vi "ADIS16470 Status.vi"(8 "error in (no error)":errorcluster, 11 "ADIS16470DevRef":T1) -> (0 "error out":errorcluster, 2 "ADIS16470 Status":T6, 3 "ADIS16470DevRef":T1)   [LabVIEW 2018]
uses:
  Typedef/ADIS16470 Status.ctl
  Typedef/ADIS16470 Device Reference.ctl
  Typedef/ADIS16470 Hardware Configuration.ctl
  <vilib>/Rock Robotics/WPI/SPI/WPI_SPIMode.ctl
  <vilib>/Rock Robotics/SystemInterfaces/DIO/FPGA_DIOChannel.ctl
  <vilib>/Rock Robotics/SystemInterfaces/spilib/spi_bus.ctl
  Typedef/ADIS16470 Data.ctl
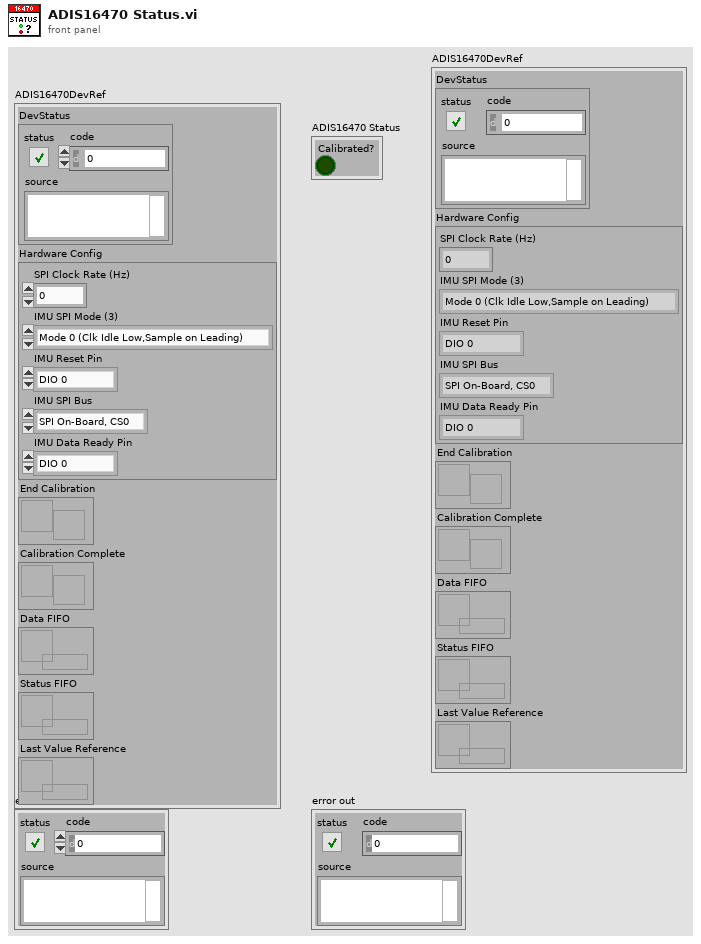
[diagram p1: front panel]
types:
  T1 = typedef "ADIS16470 Device Reference.ctl" = cluster{"DevStatus":errorcluster, "Hardware Config":T2, "End Calibration":refnum<notifier>, "Calibration Complete":refnum<notifier>, "Data FIFO":refnum<k33>, "Status FIFO":refnum<k33>, "Last Value Reference":refnum<data-value>}
  T2 = typedef "ADIS16470 Hardware Configuration.ctl" = cluster{"SPI Clock Rate (Hz)":dbl, "IMU SPI Mode (3)":T3, "IMU Reset Pin":T4, "IMU SPI Bus":T5, "IMU Data Ready Pin":T4}
  T3 = typedef "WPI_SPIMode.ctl" = enum16{"Mode 0 (Clk Idle Low,Sample on Leading)", "Mode 1 (Clk Idle Low,Sample on Trailing)", "Mode 2 (Clk Idle High,Sample on Leading)", "Mode 3 (Clk Idle High,Sample on Trailing)"}
  T4 = typedef "FPGA_DIOChannel.ctl" = enum8{"DIO 0", "DIO 1", "DIO 2", "DIO 3", "DIO 4", "DIO 5", "DIO 6", "DIO 7", "DIO 8", "DIO 9", "DIO MXP 0", "DIO MXP 1", "DIO MXP 2", "DIO MXP 3", "DIO MXP 4", "DIO MXP 5", "DIO MXP 6", "DIO MXP 7", "DIO MXP 8", "DIO MXP 9", "DIO MXP 10", "DIO MXP 11", "DIO MXP 12", "DIO MXP 13", "DIO MXP 14", "DIO MXP 15", "SPI Port CS1", "SPI Port CS2", "SPI Port CS3", "SPI Port MISO", "SPI Port MOSI", "Invalid"}
  T5 = typedef "spi_bus.ctl" = enum16{"SPI On-Board, CS0", "SPI On-Board, CS1", "SPI On-Board, CS2", "SPI On-Board, CS3", "SPI MXP", "Invalid"}
  T6 = typedef "ADIS16470 Status.ctl" = cluster{"Calibrated?":bool}
  T7 = typedef "ADIS16470 Data.ctl" = cluster{"Yaw":dbl, "Timestamp":dbl}
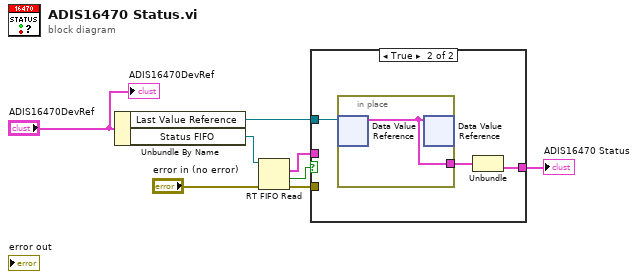
[diagram p0: block diagram]
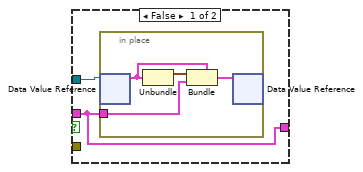
[diagram p2: hidden frame]
diagram:
  n1 = Unbundle By Name("ADIS16470DevRef") -> ("Last Value Reference"=w2:refnum<data-value>, "Status FIFO"=w7:refnum<k33>)
  n2 = RT FIFO Read(0:w7, 3:"error in (no error)") -> (9:w3:T6, 10:w5:bool, 11:w4:errorcluster)  [unwired: 2 in, 2 out]
  n3 = case shown="True" w5 {
    tunnel: w4 -> [_ _]
    tunnel: w3 -> [w9 _]
    tunnel: w2 -> [w10 w17]
    tunnel: [w9 w15] -> w1
    frame False {
      n4 = in-place {
        in-place-border: w9 -> [w11]
        n5 = in-place-dvr #1(w10) -> (w13:cluster{T7, T6})  [unwired: 1 out]
        n6 = Unbundle(w13) -> (w12:T7)  [unwired: 1 out]
        n7 = Bundle(cluster=w13, w12, w11) -> (w14:cluster{T7, T6})
        n8 = in-place-dvr #1(w14) -> ()  [unwired: 2 out]
      }
    }
    frame True {
      n9 = in-place {
        in-place-border: [w18] -> w16
        n10 = in-place-dvr #2(w17) -> (w18:cluster{T7, T6})  [unwired: 1 out]
        n11 = in-place-dvr #2(w18) -> ()  [unwired: 2 out]
      }
      n12 = Unbundle(w16) -> (w15:T6)  [unwired: 1 out]
    }
  }
  "ADIS16470 Status" <- w1
  "ADIS16470DevRef" <- "ADIS16470DevRef"
